vi "Decorations - Change Color.vi"(8 "error in (no error)":errorcluster, 10 "Decoration Color":u32(colorbox)=15224622, 11 "VI Refnum":refnum<vi>) -> (0 "error out":errorcluster, 3 "dup VI Refnum":refnum<vi>)   [LabVIEW 2017]
doc: "Dynamically changes the foreground and background colors of all Decorations, droppped from the Custom Controls palette, on the specified <b>VI Refunum</b> Front Panel to the <b>Decoration Color</b>. This VI handles the Label text color to make sure the text stands out from the <b>Decoration Color</b>."
uses:
  <vilib>/Analysis/baseanly.llb/Mean (DBL).vi
  <vilib>/UserTags/UserTags.lvlib
  <vilib>/Analysis/NI_AALBase.lvlib
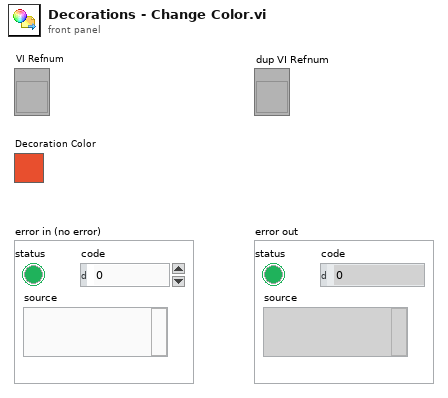
[diagram p1: front panel]
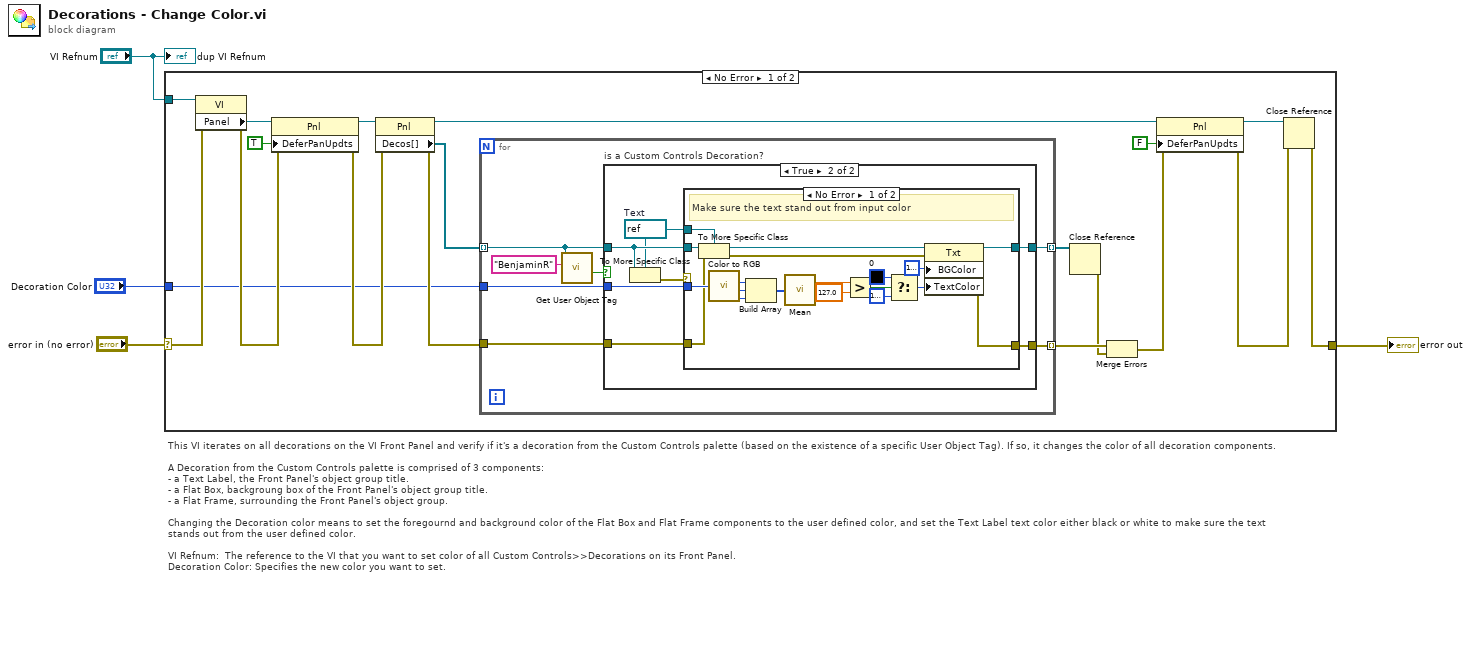
[diagram p0: block diagram]
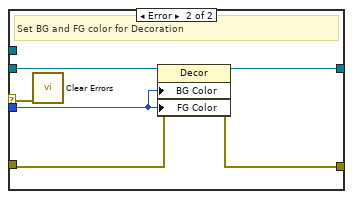
[diagram p3: hidden frame]
diagram:
  # "This VI iterates on all decorations on the VI Front Panel and verify if it's a decoration from the Custom Controls palette (based on the existence of a specific User Object Tag). If so, it changes the color of all decoration components.\n\nA Decoration from the Custom Controls palette is comprised of 3 components: \n- a Text Label, the Front Panel's object group title.\n- a Flat Box, backgroung box of the Front Panel's object group title. \n- a Flat Frame, surrounding the Front Panel's object group.\n\nChanging the Decoration color means to set the foregournd and background color of the Flat Box and Flat Frame components to the user defined color, and set the Text Label text color either black or white to make sure the text stands out from the user defined color.\n\nVI Refnum:  The reference to the VI that you want to set color of all Custom Controls>>Decorations on its Front Panel.\nDecoration Color: Specifies the new color you want to set."
  n1 = case shown="No Error" "error in (no error)" {
    selector: "error in (no error)" -> [w20 w65]
    tunnel: [w16 w65] -> w3
    tunnel: "Decoration Color" -> [w6 _]
    tunnel: "VI Refnum" -> [w5 _]
    frame No Error {
      n2 = property class="VI"(reference=w5, error in=w20) -> (error out=w13:errorcluster, "Panel"=w23:refnum<vi>)  [unwired: 1 out]
      n3 = property class="Pnl"(reference=w23, error in=w13, "DeferPanUpdts"=TRUE ("Defer Panel Updates")) -> (reference out=w15:refnum<vi>, error out=w12:errorcluster)
      n4 = property class="Pnl"(reference=w15, error in=w12) -> (reference out=w10:refnum<vi>, error out=w21:errorcluster, "Decos[]"=w22:refnum<vi>[])
      n5 = for {
        tunnel: w22 -> [w28] mode=indexing
        tunnel: w6 -> [w27]
        tunnel: [w26] -> w18 mode=indexing
        tunnel: w21 -> [w25]
        tunnel: [w24] -> w19 mode=indexing
        n6 = call <vilib>:"Get User Object Tag.vi"("Tag Name"="BenjaminR", "Generic Refnum"=w28) -> ("Was Tag Found?"=w29:bool)  [unwired: 6 in, 3 out]
        n7 = case "is a Custom Controls Decoration?" shown="True" w29 {
          tunnel: w28 -> [w32 w38]
          tunnel: w27 -> [_ w39]
          tunnel: [w32 w35] -> w26
          tunnel: w25 -> [w31 w34]
          tunnel: [w31 w33] -> w24
          frame False {
          }
          frame True {
            w36 = refnum<vi> refnum  # Text
            n8 = To More Specific Class(target class=w36, reference=w38) -> (error out=w37:errorcluster)  [unwired: 1 in, 1 out]
            n9 = case shown="No Error" w37 {
              selector: w37 -> [_ w62]
              tunnel: w39 -> [w50 w64]
              tunnel: w38 -> [w58 w63]
              tunnel: w36 -> [w57 _]
              tunnel: [w49 w61] -> w35
              tunnel: w34 -> [w48 w60]
              tunnel: [w47 w59] -> w33
              frame No Error {
                # "Make sure the text stand out from input color"
                n10 = To More Specific Class(target class=w57, reference=w58, error in=w48) -> (specific class reference=w56:refnum<vi>, error out=w55:errorcluster)
                n11 = call <vilib>:"Color to RGB.vi"("Color"=w50) -> ("R"=w44:u8, "G"=w43:u8, "B"=w42:u8)  [unwired: 1 out]
                n12 = Build Array(w44, w43, w42) -> (w41:u8[])
                n13 = call-poly <vilib>:"Mean.vi"("X"=w41) -> ("mean"=w40:dbl)  [unwired: 1 out]
                n14 = Greater?(x=w40, y=127.0) -> (0:w54:bool)
                n15 = Select(t=u32 0, s=w54, f=u32 16777226) -> (s? t:f=w46:u32)
                n16 = property class="Txt"(reference=w56, error in=w55, "BGColor"=u32 16777216 ("Text Colors:BG Color"), "TextColor"=w46) -> (reference out=w49:refnum<vi>, error out=w47:errorcluster)
              }
              frame Error {
                # "Set BG and FG color for Decoration"
                n17 = call <vilib>:"Clear Errors.vi"("error in (no error)"=w62) -> ()  [unwired: 5 in, 2 out]
                n18 = property class="Decor"(reference=w63, error in=w60, "BG Color"=w64, "FG Color"=w64) -> (reference out=w61:refnum<vi>, error out=w59:errorcluster)
              }
            }
          }
        }
      }
      n19 = Close Reference(reference=w18) -> (error out=w17:errorcluster)  [unwired: 1 in]
      n20 = Merge Errors(w19, w17) -> (w8:errorcluster)
      n21 = property class="Pnl"(reference=w10, error in=w8, "DeferPanUpdts"=FALSE ("Defer Panel Updates")) -> (reference out=w9:refnum<vi>, error out=w7:errorcluster)
      n22 = Close Reference(reference=w9, error in (no error)=w7) -> (error out=w16:errorcluster)
    }
    frame Error {
    }
  }
  "error out" <- w3
  "dup VI Refnum" <- "VI Refnum"
